vi "LoadMPCMatrix_to_mem_sim.vi"(8 "nuN_mpc":u16, 9 "Ns":u16, 11 "big_mat_data":fxp<+/-,32,3>[](array[numeric])=[0.0, 0.0, 0.0, 0.0, 0.0, 0.0, 0.0, 0.0, 0.0, 0.0, 0.0, 0.0]) -> ()   [LabVIEW 2017]
uses:
  fixed-point/typeDefs/QP_mem_type.ctl
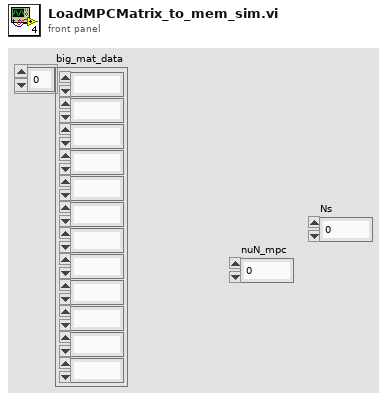
[diagram p1: front panel]
types:
  T1 = typedef "QP_mem_type.ctl" = refnum<k21>
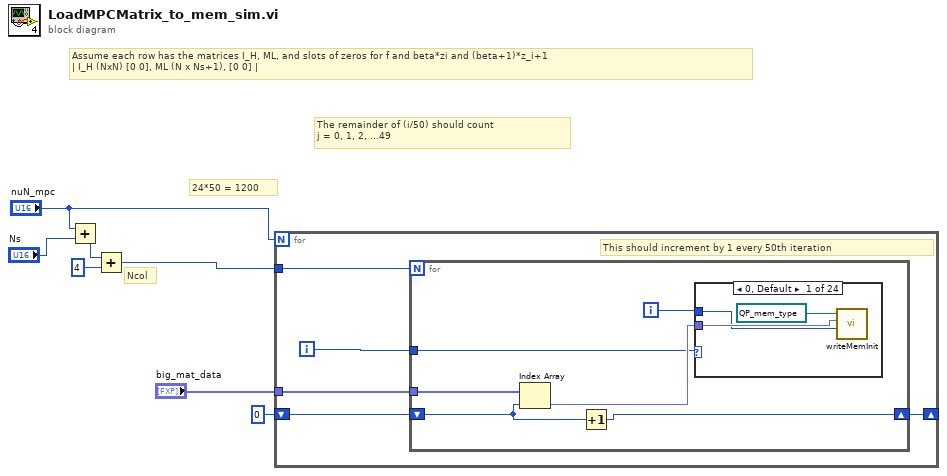
[diagram p0: block diagram]
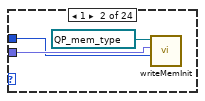
[diagram p2: hidden frame]
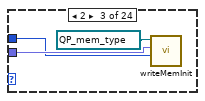
[diagram p3: hidden frame]
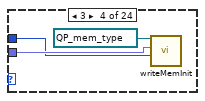
[diagram p4: hidden frame]
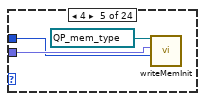
[diagram p5: hidden frame]
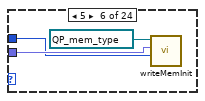
[diagram p6: hidden frame]
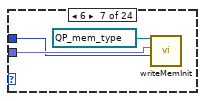
[diagram p7: hidden frame]
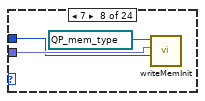
[diagram p8: hidden frame]
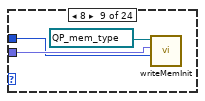
[diagram p9: hidden frame]
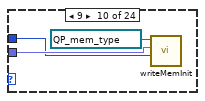
[diagram p10: hidden frame]
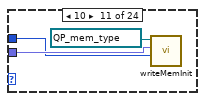
[diagram p11: hidden frame]
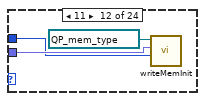
[diagram p12: hidden frame]
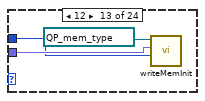
[diagram p13: hidden frame]
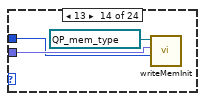
[diagram p14: hidden frame]
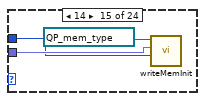
[diagram p15: hidden frame]
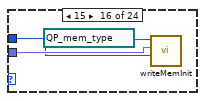
[diagram p16: hidden frame]
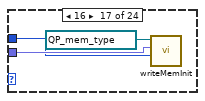
[diagram p17: hidden frame]
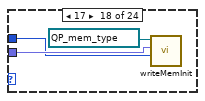
[diagram p18: hidden frame]
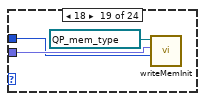
[diagram p19: hidden frame]
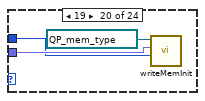
[diagram p20: hidden frame]
diagram:
  # "The remainder of (i/50) should count\nj = 0, 1, 2, ...49"
  # "Assume each row has the matrices I_H, ML, and slots of zeros for f and beta*zi and (beta+1)*z_i+1\n| I_H (NxN) [0 0], ML (N x Ns+1), [0 0] |"
  # "Ncol"
  # "24*50 = 1200"
  n1 = Add(x="nuN_mpc", y="Ns") -> (x+y=w5:u16)
  n2 = Add(x=w5, y=u16 4) -> (x+y=w1:u16)
  n3 = for {
    N: "nuN_mpc" -> [_]
    shift-right: [w9] -> _
    shift-left: u16 0 -> [w10]
    tunnel: "big_mat_data" -> [w12]
    tunnel: w1 -> [w11]
    i -> [w8]
    # "This should increment by 1 every 50th iteration"
    n4 = for {
      N: w11 -> [_]
      tunnel: w12 -> [w18]
      shift-right: [w14] -> w9
      shift-left: w10 -> [w15]
      tunnel: w8 -> [w13]
      i -> [w16]
      n5 = Index Array(array=w18, index=w15) -> (element=w17:fxp<+/-,32,3>)
      n6 = Increment(x=w15) -> (x+1=w14:u16)
      n7 = case shown="0, Default" w13 {
        tunnel: w17 -> [w21 w24 w27 w30 w33 w36 w39 w42 w45 w48 w51 w54 w57 w60 w63 w66 w69 w72 w75 w78 w81 w84 w87 w90]
        tunnel: w16 -> [w20 w23 w26 w29 w32 w35 w38 w41 w44 w47 w50 w53 w56 w59 w62 w65 w68 w71 w74 w77 w80 w83 w86 w89]
        frame 0, Default {
          n8 = call "writeMemInit.vi"("address"=w20, "data"=w21, "QP-Memory In"=T1 "Memory") -> ()  [unwired: 9 in]
        }
        frame 1 {
          n9 = call "writeMemInit.vi"("address"=w23, "data"=w24, "QP-Memory In"=T1 "Memory 2") -> ()  [unwired: 9 in]
        }
        frame 2 {
          n10 = call "writeMemInit.vi"("address"=w26, "data"=w27, "QP-Memory In"=T1 "Memory 3") -> ()  [unwired: 9 in]
        }
        frame 3 {
          n11 = call "writeMemInit.vi"("address"=w29, "data"=w30, "QP-Memory In"=T1 "Memory 4") -> ()  [unwired: 9 in]
        }
        frame 4 {
          n12 = call "writeMemInit.vi"("address"=w32, "data"=w33, "QP-Memory In"=T1 "Memory 5") -> ()  [unwired: 9 in]
        }
        frame 5 {
          n13 = call "writeMemInit.vi"("address"=w35, "data"=w36, "QP-Memory In"=T1 "Memory 6") -> ()  [unwired: 9 in]
        }
        frame 6 {
          n14 = call "writeMemInit.vi"("address"=w38, "data"=w39, "QP-Memory In"=T1 "Memory 7") -> ()  [unwired: 9 in]
        }
        frame 7 {
          n15 = call "writeMemInit.vi"("address"=w41, "data"=w42, "QP-Memory In"=T1 "Memory 8") -> ()  [unwired: 9 in]
        }
        frame 8 {
          n16 = call "writeMemInit.vi"("address"=w44, "data"=w45, "QP-Memory In"=T1 "Memory 9") -> ()  [unwired: 9 in]
        }
        frame 9 {
          n17 = call "writeMemInit.vi"("address"=w47, "data"=w48, "QP-Memory In"=T1 "Memory 10") -> ()  [unwired: 9 in]
        }
        frame 10 {
          n18 = call "writeMemInit.vi"("address"=w50, "data"=w51, "QP-Memory In"=T1 "Memory 11") -> ()  [unwired: 9 in]
        }
        frame 11 {
          n19 = call "writeMemInit.vi"("address"=w53, "data"=w54, "QP-Memory In"=T1 "Memory 12") -> ()  [unwired: 9 in]
        }
        frame 12 {
          n20 = call "writeMemInit.vi"("address"=w56, "data"=w57, "QP-Memory In"=T1 "Memory 13") -> ()  [unwired: 9 in]
        }
        frame 13 {
          n21 = call "writeMemInit.vi"("address"=w59, "data"=w60, "QP-Memory In"=T1 "Memory 14") -> ()  [unwired: 9 in]
        }
        frame 14 {
          n22 = call "writeMemInit.vi"("address"=w62, "data"=w63, "QP-Memory In"=T1 "Memory 15") -> ()  [unwired: 9 in]
        }
        frame 15 {
          n23 = call "writeMemInit.vi"("address"=w65, "data"=w66, "QP-Memory In"=T1 "Memory 16") -> ()  [unwired: 9 in]
        }
        frame 16 {
          n24 = call "writeMemInit.vi"("address"=w68, "data"=w69, "QP-Memory In"=T1 "Memory 17") -> ()  [unwired: 9 in]
        }
        frame 17 {
          n25 = call "writeMemInit.vi"("address"=w71, "data"=w72, "QP-Memory In"=T1 "Memory 18") -> ()  [unwired: 9 in]
        }
        frame 18 {
          n26 = call "writeMemInit.vi"("address"=w74, "data"=w75, "QP-Memory In"=T1 "Memory 19") -> ()  [unwired: 9 in]
        }
        frame 19 {
          n27 = call "writeMemInit.vi"("address"=w77, "data"=w78, "QP-Memory In"=T1 "Memory 20") -> ()  [unwired: 9 in]
        }
        frame 20 {
          n28 = call "writeMemInit.vi"("address"=w80, "data"=w81, "QP-Memory In"=T1 "Memory 21") -> ()  [unwired: 9 in]
        }
        frame 21 {
          n29 = call "writeMemInit.vi"("address"=w83, "data"=w84, "QP-Memory In"=T1 "Memory 22") -> ()  [unwired: 9 in]
        }
        frame 22 {
          n30 = call "writeMemInit.vi"("address"=w86, "data"=w87, "QP-Memory In"=T1 "Memory 23") -> ()  [unwired: 9 in]
        }
        frame 23 {
          n31 = call "writeMemInit.vi"("address"=w89, "data"=w90, "QP-Memory In"=T1 "Memory 24") -> ()  [unwired: 9 in]
        }
      }
    }
  }
